vi "streamWrite.vi"(8 "error in (no error)":errorcluster, 9 "Front of stream":bool, 10 "String":string, 11 "TextTestRunner in":refnum<class "TextTestRunner.lvclass">) -> (0 "error out":errorcluster, 3 "TextTestRunner out":refnum<class "TextTestRunner.lvclass">)   [LabVIEW 2013, in "TextTestRunner.lvclass"]
uses:
  TextTestRunner.lvclass
  TextTestRunner.lvclass/TextTestRunner.ctl
panel:
  # "JKI VI Tester for LabVIEW\nhttp://jkisoft.com/vi-tester\nCopyright (C) 2007-2009, JKI <info@jkisoft.com>\nALL RIGHTS RESERVED"
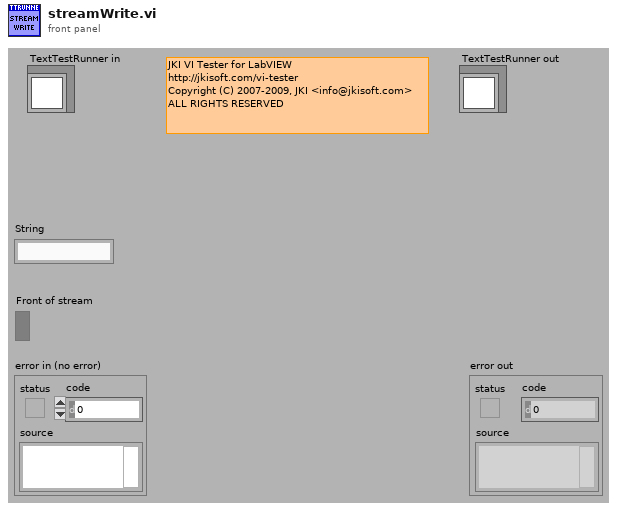
[diagram p1: front panel]
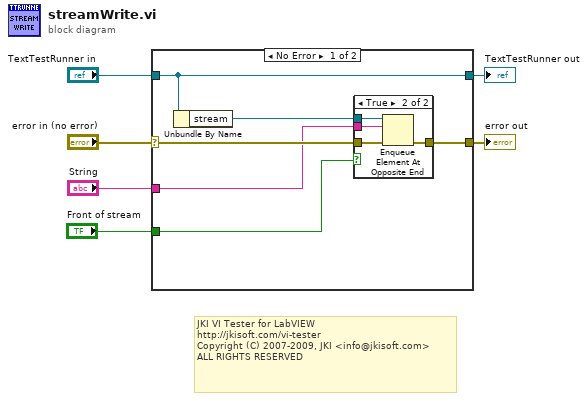
[diagram p0: block diagram]
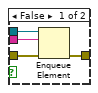
[diagram p2: hidden frame]
diagram:
  # "JKI VI Tester for LabVIEW\nhttp://jkisoft.com/vi-tester\nCopyright (C) 2007-2009, JKI <info@jkisoft.com>\nALL RIGHTS RESERVED"
  n1 = case shown="No Error" "error in (no error)" {
    selector: "error in (no error)" -> [w10 w22]
    tunnel: [w9 w22] -> w5
    tunnel: [w12 w21] -> w3
    tunnel: "TextTestRunner in" -> [w12 w21]
    tunnel: "String" -> [w8 _]
    tunnel: "Front of stream" -> [w7 _]
    frame No Error {
      n2 = Unbundle By Name(w12) -> ("stream"=w11:refnum<queue>)
      n3 = case shown="True" w7 {
        tunnel: w11 -> [w16 w20]
        tunnel: w10 -> [w15 w18]
        tunnel: [w14 w17] -> w9
        tunnel: w8 -> [w13 w19]
        frame False {
          n4 = Enqueue Element(queue=w16, element=w13, error in (no error)=w15) -> (error out=w14:errorcluster)  [unwired: 1 in, 2 out]
        }
        frame True {
          n5 = Enqueue Element At Opposite End(queue=w20, element=w19, error in (no error)=w18) -> (error out=w17:errorcluster)  [unwired: 1 in, 2 out]
        }
      }
    }
    frame Error {
    }
  }
  "error out" <- w5
  "TextTestRunner out" <- w3
